vi "Save picture camera.vi"() -> ()   [LabVIEW 2015]
panel:
  in  "Save Picture Camera":bool
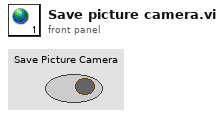
[diagram p1: front panel]
diagram:
